vi "Configure Range.vi"(7 "Auto Range (T: Enable)":bool=TRUE, 8 "error in (no error)":errorcluster, 9 "Lower Limit (-90.0 dBm)":dbl=-90.0 format="%#.6g", 10 "Upper Limit (90.0 dBm)":dbl=90.0 format="%#.6g", 11 "VISA resource name":refnum<visa-resource-name>) -> (0 "error out":errorcluster, 3 "VISA resource name out":refnum<visa-resource-name>)   [LabVIEW 2015, in "Template - Power Meter.lvlib"]
doc: "Configures the instrument's ranging capabilities. Enabling auto ranging allows the instrument to choose its own range. Otherwise, custom limits can be used to set up the range. Should the range be exceeded, the result can be known by calling the <b>Query Range Test</b> VI."
uses:
  <instrlib>/_Template - Power Meter/Template - Power Meter.lvlib
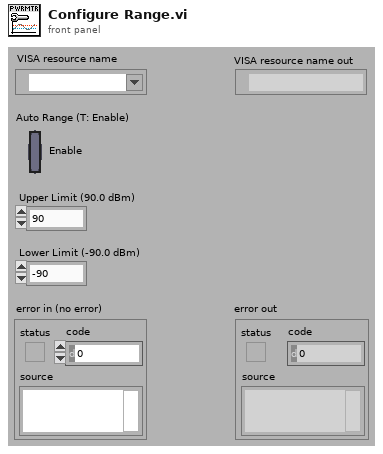
[diagram p1: front panel]
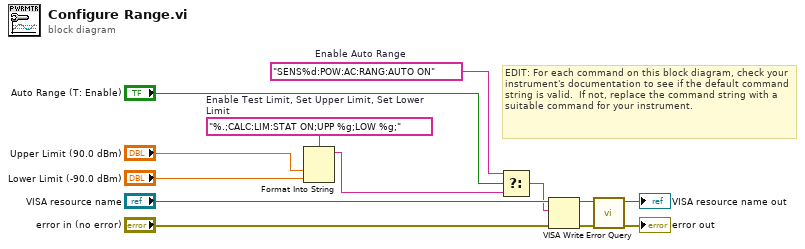
[diagram p0: block diagram]
diagram:
  w3 = "SENS%d:POW:AC:RANG:AUTO ON"  # Enable Auto Range
  w5 = "%.;CALC:LIM:STAT ON;UPP %g;LOW %g;"  # Enable Test Limit, Set Upper Limit, Set Lower Limit
  # "EDIT: For each command on this block diagram, check your instrument's documentation to see if the default command string is valid.  If not, replace the command string with a suitable command for your instrument."
  n1 = Format Into String(format string=w5, "Upper Limit (90.0 dBm)", "Lower Limit (-90.0 dBm)") -> (resulting string=w2:string)  [unwired: 2 in, 1 out]
  n2 = Select(t=w3, s="Auto Range (T: Enable)", f=w2) -> (s? t:f=w4:string)
  n3 = VISA Write(VISA resource name="VISA resource name", write buffer=w4, error in (no error)="error in (no error)") -> (VISA resource name out=w11:refnum<visa-resource-name>, error out=w9:errorcluster)  [unwired: 1 out]
  n4 = call <instrlib>:"Error Query.vi"("error in (no error)"=w9, "VISA resource name"=w11) -> ("error out"=→"error out":errorcluster, "VISA resource name out"=→"VISA resource name out":refnum<visa-resource-name>)  [unwired: 6 in, 2 out]
